vi "Cable Tester Front.vi"() -> ()   [LabVIEW 2012]
panel:
  out "Channel 16 (AI 23)":dynamicdata(graph)
  out "Channel 15 (AI 22)":dynamicdata(graph)
  out "Channel 14 (AI 21)":dynamicdata(graph)
  out "Channel 13 (AI 20)":dynamicdata(graph)
  out "Channel 12 (AI 19)":dynamicdata(graph)
  out "Channel 11 (AI 18)":dynamicdata(graph)
  out "Channel 10 (AI 17)":dynamicdata(graph)
  out "Channel 9 (AI 16)":dynamicdata(graph)
  out "Channel 4 (AI 3)":dynamicdata(graph)
  out "Channel 8 (AI 7)":dynamicdata(graph)
  out "Channel 7 (AI 6)":dynamicdata(graph)
  out "Channel 3 (AI 2)":dynamicdata(graph)
  out "Channel 2 (AI 1)":dynamicdata(graph)
  out "Channel 5 (AI 4)":dynamicdata(graph)
  out "Channel 6 (AI 5)":dynamicdata(graph)
  out "Channel 1 (AI 0)":dynamicdata(graph)
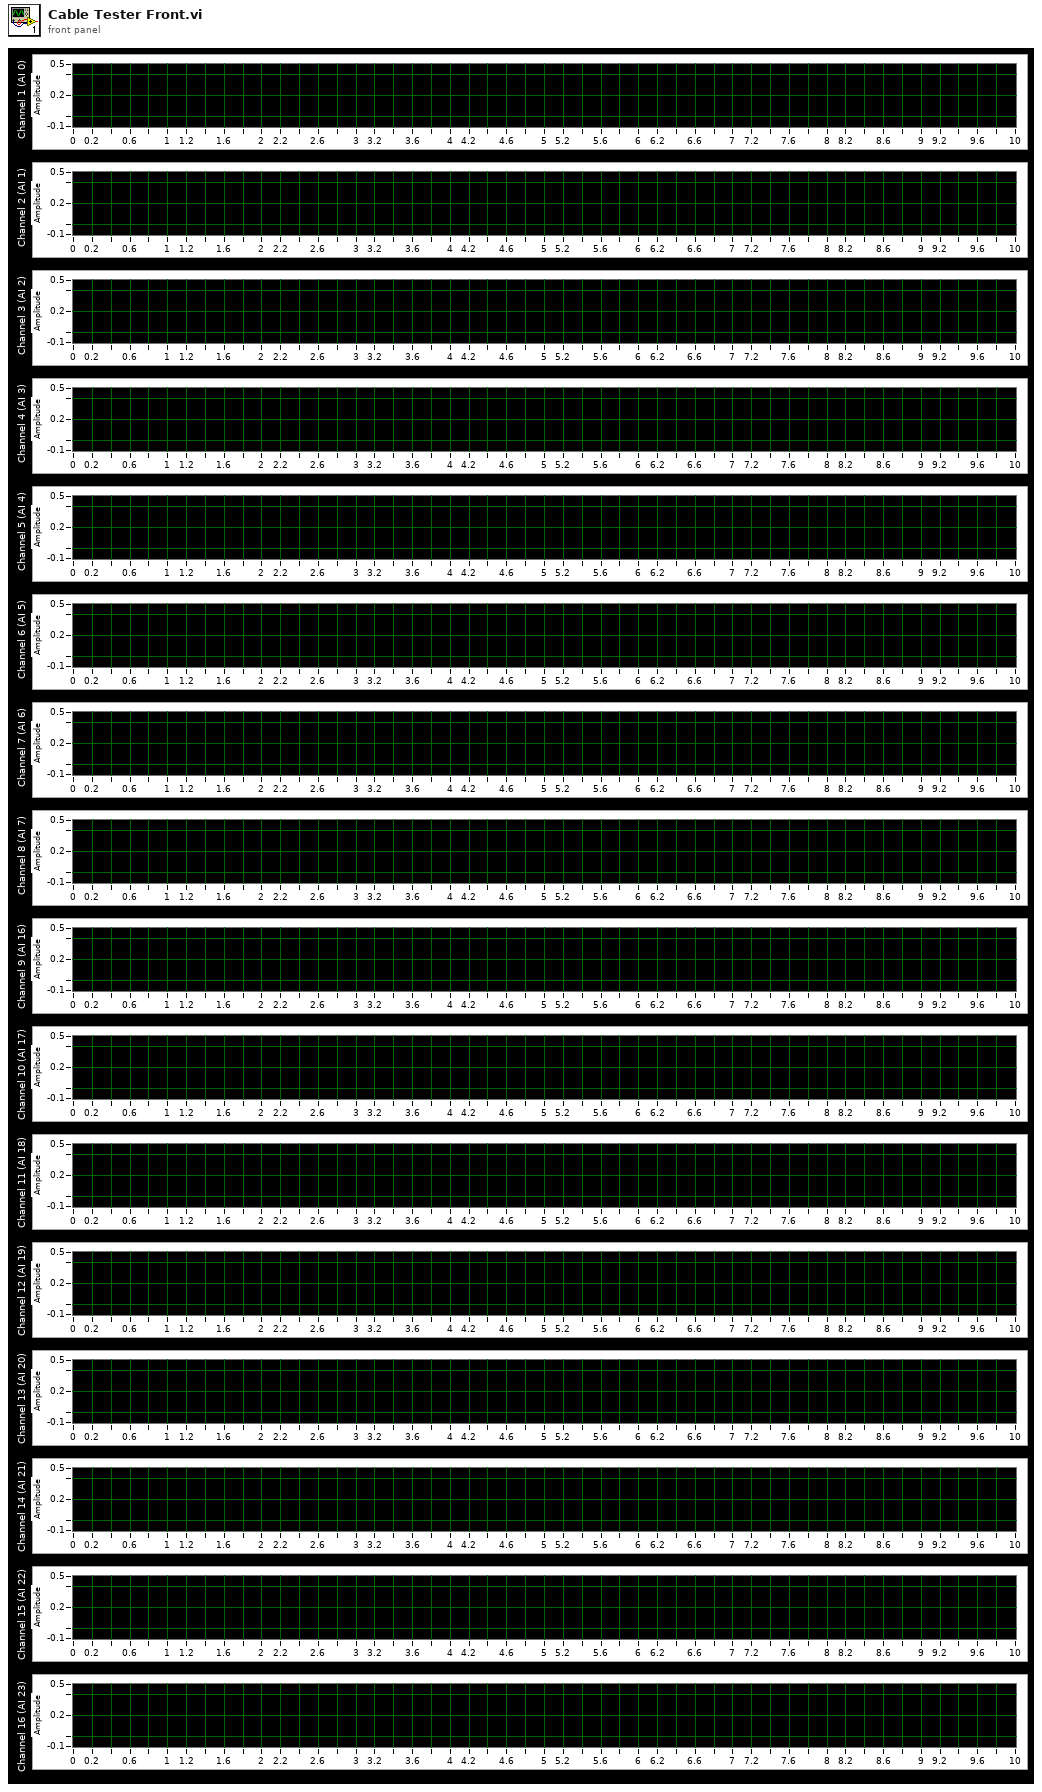
[diagram p1: front panel]
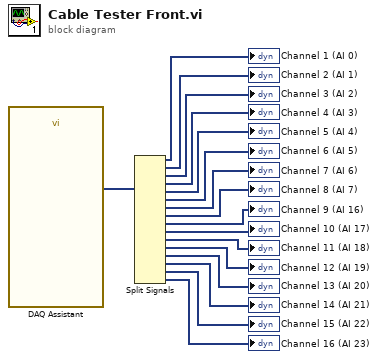
[diagram p0: block diagram]
diagram:
  n1 = call "DAQ Assistant"() -> ("data"=w17:dynamicdata)  [unwired: 17 in, 2 out]
  n2 = Split Signals(w17) -> (→"Channel 1 (AI 0)":dynamicdata, →"Channel 2 (AI 1)":dynamicdata, →"Channel 3 (AI 2)":dynamicdata, →"Channel 4 (AI 3)":dynamicdata, →"Channel 5 (AI 4)":dynamicdata, →"Channel 6 (AI 5)":dynamicdata, →"Channel 7 (AI 6)":dynamicdata, →"Channel 8 (AI 7)":dynamicdata, →"Channel 9 (AI 16)":dynamicdata, →"Channel 10 (AI 17)":dynamicdata, →"Channel 11 (AI 18)":dynamicdata, →"Channel 12 (AI 19)":dynamicdata, →"Channel 13 (AI 20)":dynamicdata, →"Channel 14 (AI 21)":dynamicdata, →"Channel 15 (AI 22)":dynamicdata, →"Channel 16 (AI 23)":dynamicdata)  [unwired: 16 in]
